vi "Actor Core.vi"(8 "error in":errorcluster, 11 "RandomDataChart in":refnum<class "MultiSubscriber.lvclass">) -> (0 "error out":errorcluster, 3 "Actor out":refnum<class "Actor.lvclass">)   [LabVIEW 2015, in "TestViewables.lvlib" / "MultiSubscriber.lvclass"]
doc: "(<B>Filename</B>: Actor Framework.lvlib:Actor.lvclass:Actor Core.vi)\n\nReceives messages to the actor, reacts to them, and initiates any error handling that may shut the actor down.\n\nDescendant classes may override this VI to append parallel tasks for the actor to complete while it handles messages. Overrides use the Call Parent Method node."
uses:
  MultiSubscriber.lvclass
  <vilib>/ActorFramework/Actor/Actor.lvclass
  MultiSubscriber Messages/Notification Msg/UpdateChart Msg.lvclass
  MultiSubscriber.lvclass/MultiSubscriber.ctl
  Framework/IViewable/IViewable/IViewable.lvclass
  Framework/IObserver/IObserver/IObserver.lvclass
panel:
  in  "Bound by Caption":dbl caption="Random Number"
  out "Random Percentage":dbl(graph)
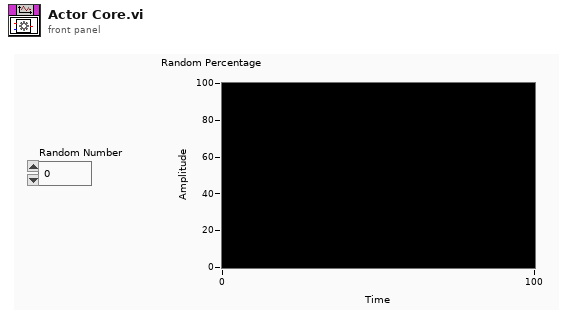
[diagram p1: front panel]
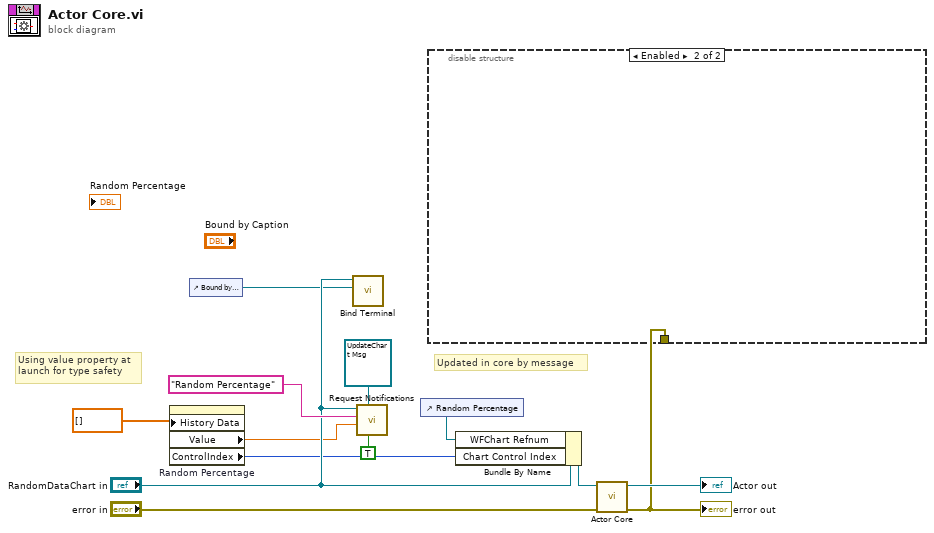
[diagram p0: block diagram]
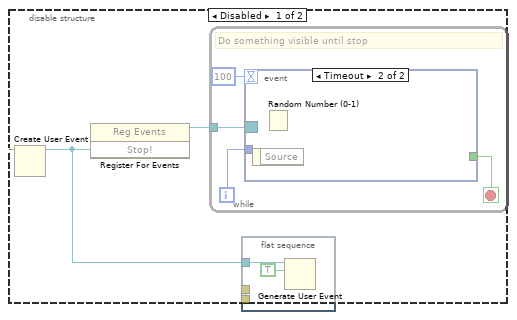
[diagram p2: hidden frame]
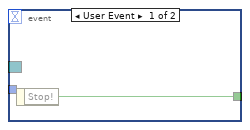
[diagram p3: hidden frame]
diagram:
  # "Using value property at\nlaunch for type safety"
  # "Updated in core by message"
  n1 = property on="Random Percentage" class="WFChart (strict)"("History Data"=dbl[] []) -> ("Value"=w6:dbl, "ControlIndex"=w7:i32)  [unwired: 2 in, 2 out]
  n2 = control-ref of="Bound by Caption"() -> (w9:refnum<vi>)
  n3 = call "Bind Terminal.vi"("Ctl Refnum"=w9, "IObserver in"="RandomDataChart in") -> ()  [unwired: 8 in, 2 out]
  n4 = call "Request Notifications.vi"("Value Changes Only? (T)"=TRUE ("Value Changes Only? (F)"), "Notification Msg (Type)"=refnum<class "UpdateChart Msg.lvclass"> refnum ("TestActors.lvlib:MultiSubscriberNotification Msg.lvclass"), "Data Type"=w6, "Topic Name"="Random Percentage", "IObserver in"="RandomDataChart in") -> ()  [unwired: 5 in, 2 out]
  n5 = control-ref of="Random Percentage"() -> (w5:refnum<vi>)
  n6 = Bundle By Name(cluster="RandomDataChart in", "WFChart Refnum"=w5, "Chart Control Index"=w7) -> (w8:refnum<class "MultiSubscriber.lvclass">)
  n7 = call-parent "Actor Core.vi"("error in"="error in", "IViewable In"=w8) -> ("error out"=w4:errorcluster, "Actor out"=→"Actor out":refnum<class "Actor.lvclass">)  [unwired: 8 in]
  "error out" <- w4
  n8 = disable-structure shown="Enabled" {
    disable-tunnel: w4 -> [w14 _]
    frame Disabled {
      w16 = FALSE  # Stop!
      n9 = Create User Event(user event datatype=w16) -> (user event=w15:refnum<user-event>)  [unwired: 1 in, 1 out]
      n10 = register-events(w15) -> (reference out=w17:refnum<event-registration>)  [unwired: 2 in, 1 out]
      n11 = while {
        tunnel: w17 -> [w23]
        i -> [w21]
        stop <- w22 stop-if-true
        # "Do something visible until stop"
        n12 = event shown="[1] Timeout" {
          selector: w23 -> [_ _]
          dyn-events: _ -> [_ _]
          timeout: 100 -> [_ _]
          tunnel: [w24 _] -> w22
          tunnel: w21 -> [_ _]
          event User Event {
            n13 = event-data() -> ("Stop!"=w24:bool)  [unwired: 1 in]
          }
          event Timeout {
            n14 = event-data() -> ()  [unwired: 1 in, 1 out]
            n15 = Random Number (0-1)() -> (number: 0 to 1=w25:dbl)
          }
        }
      }
      n16 = flat-sequence {
        tunnel: w15 -> [w19]
        tunnel: w14 -> [_]
        frame #0 {
          n17 = Generate User Event(user event=w19, event data cluster=TRUE ("event data")) -> ()  [unwired: 2 in, 2 out]
        }
      }
    }
    frame Enabled {
    }
  }
